vi "estiBendingMode.vi"(7 "Truncation Threshold":dbl=0.0001, 8 "error in (no error)":errorcluster, 9 "Actuator Force (N)":dbl[](array[numeric]), 10 "Mirror":enum16{"M1M3", "M2"}(ring), 11 "BendModeToForce in":refnum<class "BendModeToForce.lvclass">) -> (0 "error out":errorcluster, 2 "Mirror DOF (um)":dbl[](array[numeric]), 3 "BendModeToForce out":refnum<class "BendModeToForce.lvclass">)   [LabVIEW 2016, in "BendModeToForce.lvclass"]
doc: "Estimate the bending mode from figure actuator forces."
uses:
  BendModeToForce.lvclass
  BendModeToForce.lvclass/BendModeToForce.ctl
  <vilib>/Analysis/_algsub.llb/Real PseudoInverse Matrix.vi
  <vilib>/Analysis/Matrix/Numeric/Conversions/Array To Matrix - RA2.vi
  <vilib>/Analysis/Matrix/Numeric/Conversions/Matrix To Array - RM.vi
  <vilib>/Analysis/NI_AALPro.lvlib
  <vilib>/Analysis/Matrix/NI_Matrix.lvlib
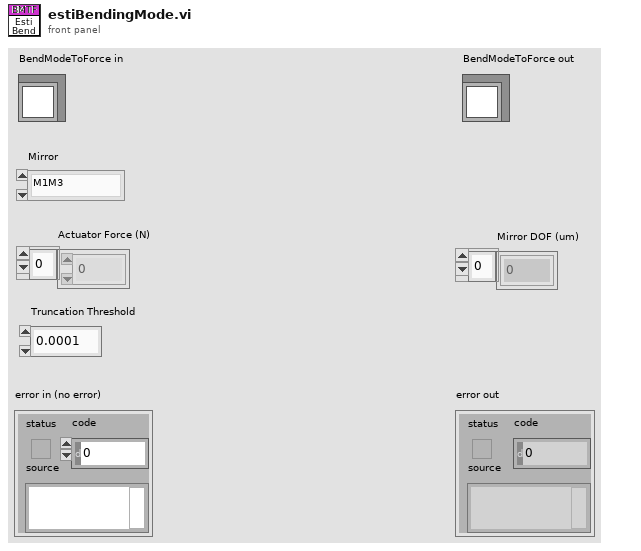
[diagram p1: front panel]
types:
  T1 = typedef "NI_Matrix.lvlib/RealMatrix.ctl" = dbl[][]
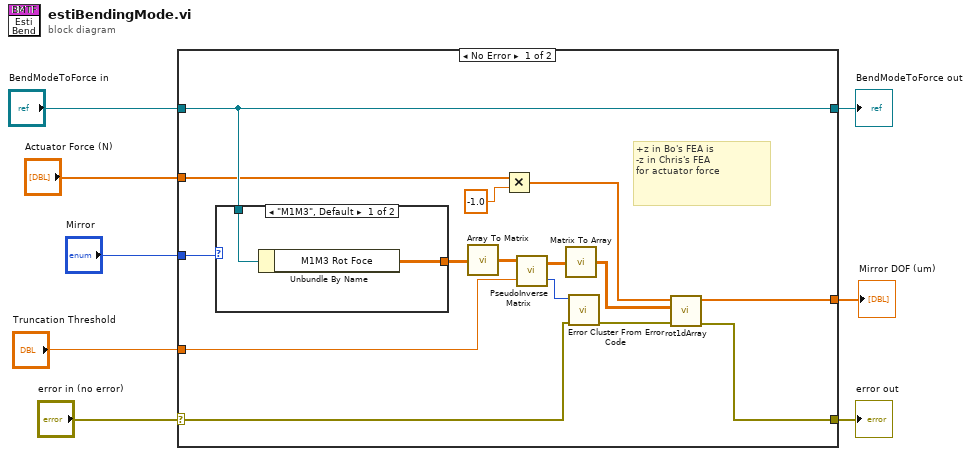
[diagram p0: block diagram]
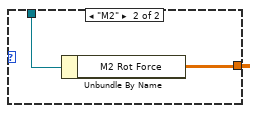
[diagram p2: hidden frame]
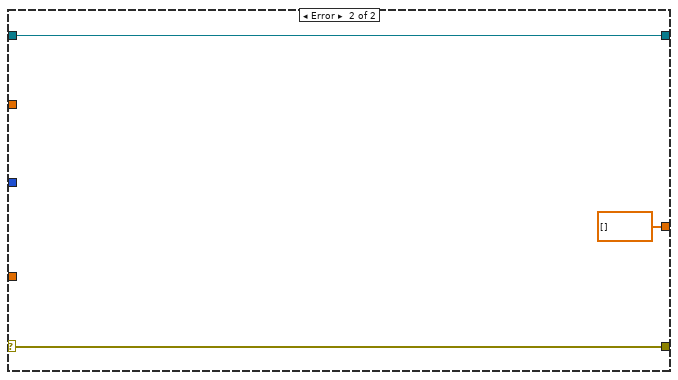
[diagram p3: hidden frame]
diagram:
  n1 = case shown="No Error" "error in (no error)" {
    selector: "error in (no error)" -> [w16 w30]
    tunnel: [w13 w30] -> w7
    tunnel: [w22 w29] -> w6
    tunnel: "BendModeToForce in" -> [w22 w29]
    tunnel: "Mirror" -> [w23 _]
    tunnel: "Truncation Threshold" -> [w19 _]
    tunnel: "Actuator Force (N)" -> [w11 _]
    tunnel: [w9 dbl[] [] ("Rotated 1D Array")] -> w2
    frame No Error {
      # "+z in Bo's FEA is \n-z in Chris's FEA\nfor actuator force"
      n2 = case shown="\"M1M3\", Default" w23 {
        tunnel: w22 -> [w25 w27]
        tunnel: [w24 w26] -> w21
        frame "M1M3", Default {
          n3 = Unbundle By Name(w25) -> ("M1M3 Rot Foce"=w24:dbl[][])
        }
        frame "M2" {
          n4 = Unbundle By Name(w27) -> ("M2 Rot Force"=w26:dbl[][])
        }
      }
      n5 = call-poly <vilib>:"Array To Matrix.vi"("Real 2D Array"=w21) -> ("Real Matrix"=w20:T1)
      n6 = Multiply(x=w11, y=-1.0) -> (x*y=w10:dbl[])
      n7 = call-poly <vilib>:"PseudoInverse Matrix.vi"("tolerance"=w19, "Input Matrix"=w20) -> ("error"=w17:i32, "PseudoInverse Matrix"=w18:T1)
      n8 = call-poly <vilib>:"Matrix To Array.vi"("Real Matrix"=w18) -> ("Real 2D Array"=w12:dbl[][])
      n9 = call <vilib>:"Error Cluster From Error Code.vi"("error in (no error)"=w16, "error code (0)"=w17) -> ("error out"=w14:errorcluster)  [unwired: 7 in]
      n10 = call "rot1dArray.vi"("error in (no error)"=w14, "Rot Mat"=w12, "1D Array"=w10) -> ("error out"=w13:errorcluster, "Rotated 1D Array"=w9:dbl[])  [unwired: 7 in]
    }
    frame Error {
    }
  }
  "error out" <- w7
  "BendModeToForce out" <- w6
  "Mirror DOF (um)" <- w2
